vi "ZAlign_Begin.vi"(0 "VI in":refnum<vi>, 5 "Undo Name":string, 7 "WithUndo":bool=TRUE, 11 "error in (no error)":errorcluster) -> (4 "VIRef":refnum<vi>, 6 "PanelRef":refnum<vi>, 8 "SelectedElements?":bool, 15 "error out":errorcluster)   [LabVIEW 2014, in "ZAlign.lvlib"]
doc: "ZAlign.lvlib:ZAlign_Begin.vi\n----------------------------------------------\nStart des Quickdrops.\n\nInputs:\n---------------------\n- VI in : Refnum; \n- Undo Name : String; \n- error in (no error) : Cluster; \n\nOutputs:\n---------------------\n- VIRef : Refnum; \n- PanelRef : Refnum; \n- SelectedElements? : Boolean; \n- error out : Cluster; \n\n----------------------------------------------\n26.03.2015 jcm\nZühlke Engineering AG\nCH-8952 Schlieren\nwww.zuehlke.com"
uses:
  ZAlign.lvlib
panel:
  # "Connector Pane"
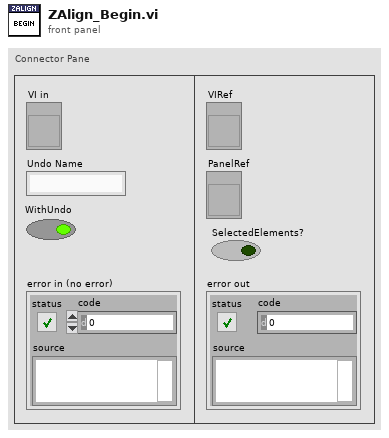
[diagram p1: front panel]
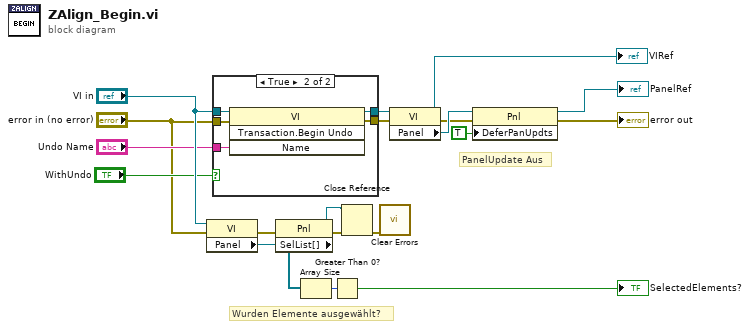
[diagram p0: block diagram]
diagram:
  # "PanelUpdate Aus"
  # "Wurden Elemente ausgewählt?"
  n1 = property class="VI"(reference="VI in", error in="error in (no error)") -> (error out=w9:errorcluster, "Panel"=w5:refnum<vi>)  [unwired: 1 out]
  n2 = case shown="True" "WithUndo" {
    tunnel: [w21 w27] -> w14
    tunnel: [w22 w26] -> w13
    tunnel: "VI in" -> [w22 w25]
    tunnel: "Undo Name" -> [_ w24]
    tunnel: "error in (no error)" -> [w21 w23]
    frame False {
    }
    frame True {
      n3 = invoke class="VI" method="Transaction.Begin Undo"(reference=w25, error in=w23, "Name"=w24) -> (reference out=w26:refnum<vi>, error out=w27:errorcluster)  [unwired: 1 in, 2 out]
    }
  }
  n4 = property class="Pnl"(reference=w5, error in=w9) -> (reference out=w11:refnum<vi>, error out=w10:errorcluster, "SelList[]"=w6:refnum<vi>[])
  n5 = Array Size(array=w6) -> (size(s)=w7:i32)
  n6 = Greater Than 0?(x=w7) -> (x > 0?=→"SelectedElements?":bool)
  n7 = Close Reference(reference=w11, error in (no error)=w10) -> (error out=w12:errorcluster)
  n8 = call <vilib>:"Clear Errors.vi"("error in (no error)"=w12) -> ()  [unwired: 5 in, 2 out]
  n9 = property class="VI"(reference=w13, error in=w14) -> (reference out=→"VIRef":refnum<vi>, error out=w15:errorcluster, "Panel"=w18:refnum<vi>)
  n10 = property class="Pnl"(reference=w18, error in=w15, "DeferPanUpdts"=TRUE ("Defer Panel Updates")) -> (reference out=→"PanelRef":refnum<vi>, error out=→"error out":errorcluster)
